vi "filter CSM States.vi"(8 "Interface-Filter":enum16{"API-Only", "UserDef States", "All"}(ring), 11 "Array":string[](array[string])) -> (3 "filtered array":string[](array[string]))   [LabVIEW 2017, in "CSM-Helper.lvclass"]
uses:
  _csmHelper/CSM-Helper.lvclass
  _Shared/CSM Shared.lvlib
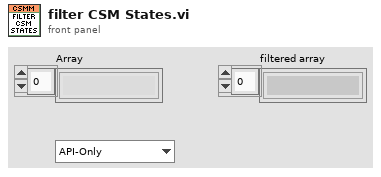
[diagram p1: front panel]
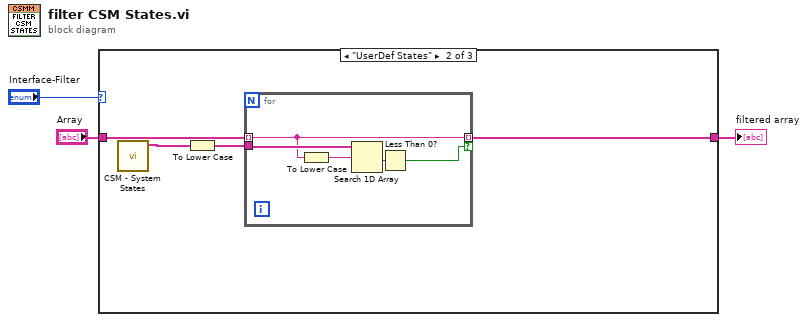
[diagram p0: block diagram]
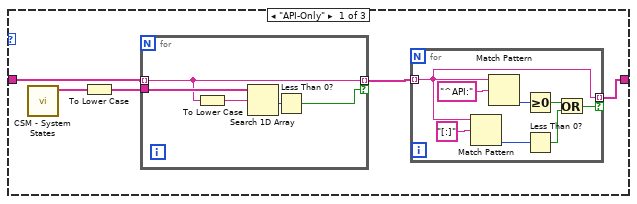
[diagram p2: hidden frame]
diagram:
  n1 = case shown="\"UserDef States\"" "Interface-Filter" {
    tunnel: [w8 w25 w31] -> w3
    tunnel: "Array" -> [w5 w24 w31]
    frame "API-Only" {
      n2 = call "CSM - System States.vi"() -> ("items to filter"=w6:string[])  [unwired: 11 in]
      n3 = To Lower Case(string=w6) -> (all lower case string=w4:string[])
      n4 = for {
        tunnel: [w12] -> w7 mode=indexing if=w10
        tunnel: w5 -> [w12] mode=indexing
        tunnel: w4 -> [w13]
        n5 = To Lower Case(string=w12) -> (all lower case string=w9:string)
        n6 = Search 1D Array(1D array=w13, element=w9) -> (index of element=w11:i32)  [unwired: 1 in]
        n7 = Less Than 0?(x=w11) -> (x < 0?=w10:bool)
      }
      n8 = for {
        tunnel: w7 -> [w17] mode=indexing
        tunnel: [w17] -> w8 mode=indexing if=w14
        n9 = Match Pattern(string=w17, regular expression="[:]") -> (offset past match=w18:i32)  [unwired: 1 in, 3 out]
        n10 = Match Pattern(string=w17, regular expression="^API:") -> (offset past match=w19:i32)  [unwired: 1 in, 3 out]
        n11 = Greater Or Equal To 0?(x=w19) -> (x >= 0?=w16:bool)
        n12 = Less Than 0?(x=w18) -> (x < 0?=w15:bool)
        n13 = Or(x=w16, y=w15) -> (x .or. y?=w14:bool)
      }
    }
    frame "UserDef States" {
      n14 = call "CSM - System States.vi"() -> ("items to filter"=w23:string[])  [unwired: 11 in]
      n15 = To Lower Case(string=w23) -> (all lower case string=w22:string[])
      n16 = for {
        tunnel: [w29] -> w25 mode=indexing if=w27
        tunnel: w24 -> [w29] mode=indexing
        tunnel: w22 -> [w30]
        n17 = To Lower Case(string=w29) -> (all lower case string=w26:string)
        n18 = Search 1D Array(1D array=w30, element=w26) -> (index of element=w28:i32)  [unwired: 1 in]
        n19 = Less Than 0?(x=w28) -> (x < 0?=w27:bool)
      }
    }
    frame "All" {
    }
  }
  "filtered array" <- w3
